vi "Save TestNameTXT.vi"(10 "Paramer Set":string[][](table), 11 "名称或相对路径":string="UserDefine.ini") -> ()   [LabVIEW 2011]
uses:
  Global System.vi
  <vilib>/Utility/file.llb/Write To Spreadsheet File (string).vi
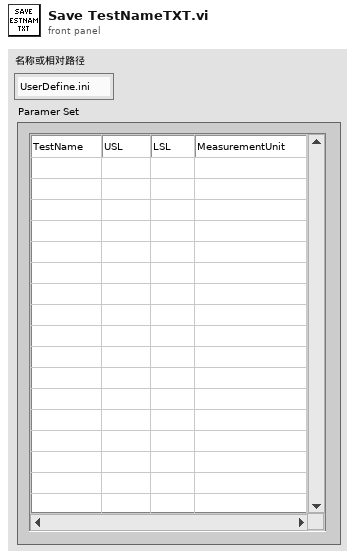
[diagram p1: front panel]
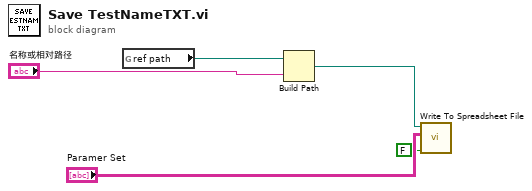
[diagram p0: block diagram]
diagram:
  n1 = global read "Global System.vi" "ref path"() -> (w5:path)
  n2 = Build Path(base path=w5, name or relative path="名称或相对路径") -> (appended path=w3:path)
  n3 = call-poly <vilib>:"Write To Spreadsheet File.vi"("append to file? (new file:F)"=FALSE, "2D data"="Paramer Set", "file path (dialog if empty)"=w3) -> ()  [unwired: 5 in, 1 out]
